vi "GrubbsTest.vi"(4 "Значимость":dbl, 6 "Исходные":dbl[](graph)) -> (0 "СКО":dbl, 1 "Среднее":dbl, 2 "Промахи":dbl[](array[numeric]), 3 "Обработанные":dbl[](graph))   [LabVIEW 2013]
uses:
  <vilib>/Analysis/NI_AALBase.lvlib
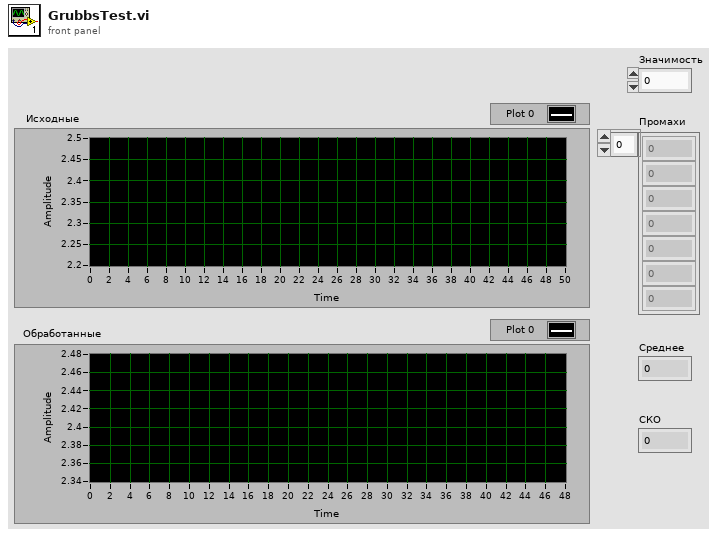
[diagram p1: front panel]
types:
  T1 = enum16{"Init", "GradeCount", "MissChecks", "fin"}
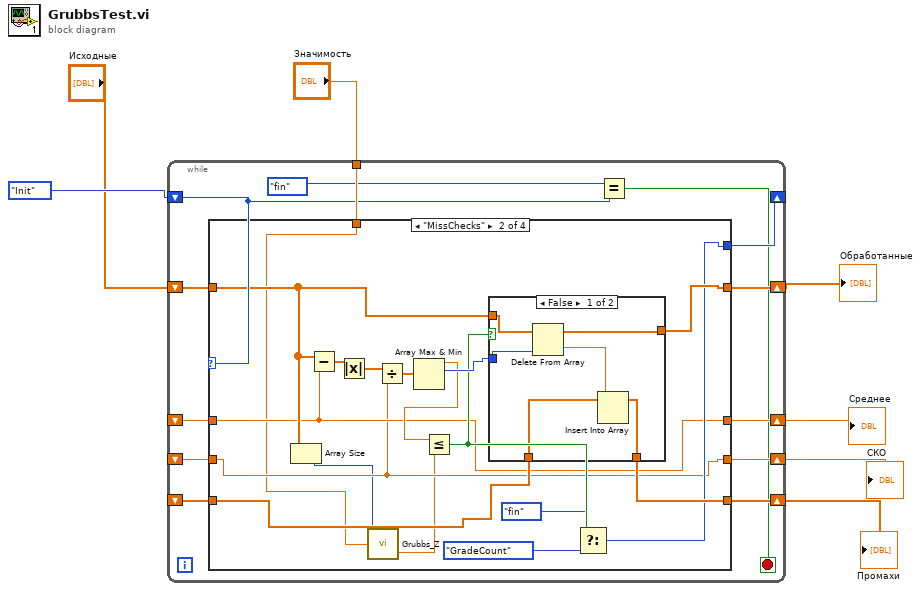
[diagram p0: block diagram]
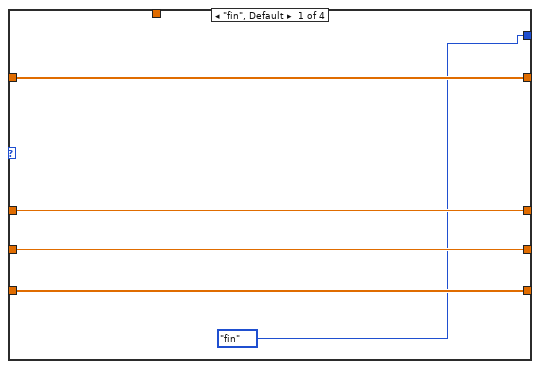
[diagram p2: hidden frame]
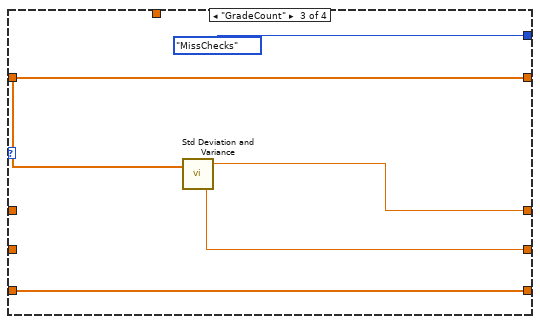
[diagram p4: hidden frame]
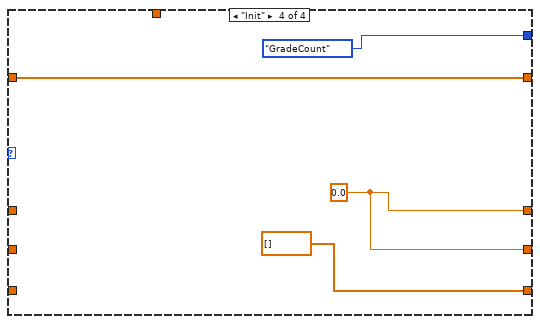
[diagram p5: hidden frame]
diagram:
  n1 = while {
    shift-right: [w20] -> _
    shift-left: T1."Init" -> [w9]
    tunnel: "Значимость" -> [w19]
    shift-right: [w14] -> w5
    shift-left: "Исходные" -> [w18]
    shift-right: [w17] -> w4
    shift-left: _ -> [w11]
    shift-right: [w16] -> w3
    shift-left: _ -> [w12]
    shift-right: [w15] -> w2
    shift-left: _ -> [w13]
    stop <- w10 stop-if-true
    n2 = case shown="\"MissChecks\"" w9 {
      tunnel: [T1."fin" w35 T1."MissChecks" T1."GradeCount"] -> w20
      tunnel: w19 -> [_ w26 _ _]
      tunnel: w18 -> [w22 w32 w55 w59]
      tunnel: [w23 w31 w54 w58] -> w17
      tunnel: [w24 w30 w56 w58] -> w16
      tunnel: [w25 w42 w53 dbl[] []] -> w15
      tunnel: [w22 w41 w55 w59] -> w14
      tunnel: w13 -> [w25 w34 w53 _]
      tunnel: w12 -> [w24 w30 _ _]
      tunnel: w11 -> [w23 w31 _ _]
      frame "fin", Default {
      }
      frame "MissChecks" {
        n3 = Array Size(array=w32) -> (size(s)=w28:i32)
        n4 = Subtract(x=w32, y=w31) -> (x-y=w33:dbl[])
        n5 = Absolute Value(x=w33) -> (abs(x)=w43:dbl[])
        n6 = call "Grubbs_Z.vi"("n"=w28, "q"=w26) -> ("G"=w27:dbl)  [unwired: 2 in]
        n7 = Divide(x=w43, y=w30) -> (x/y=w29:dbl[])
        n8 = Array Max & Min(array=w29) -> (max value=w39:dbl, max index (indices)=w40:i32)  [unwired: 2 out]
        n9 = Less Or Equal?(x=w39, y=w27) -> (x <= y?=w38:bool)
        n10 = case shown="False" w38 {
          tunnel: w32 -> [w48 w51]
          tunnel: [w45 w50] -> w42
          tunnel: [w47 w51] -> w41
          tunnel: w40 -> [w44 _]
          tunnel: w34 -> [w46 w50]
          frame False {
            n11 = Delete From Array(array=w48, index=w44) -> (deleted portion=w49:dbl, array with subset deleted=w47:dbl[])  [unwired: 1 in]
            n12 = Insert Into Array(array=w46, new element=w49) -> (w45:dbl[])  [unwired: 1 in]
          }
          frame True {
          }
        }
        n13 = Select(t=T1."fin", s=w38, f=T1."GradeCount") -> (s? t:f=w35:T1)
      }
      frame "GradeCount" {
        n14 = call <vilib>:"Std Deviation and Variance.vi"("X"=w55) -> ("mean"=w54:dbl, "standard deviation"=w56:dbl)  [unwired: 1 in, 1 out]
      }
      frame "Init" {
        w58 = 0.0
      }
    }
    n15 = Equal?(x=T1."fin", y=w9) -> (x = y?=w10:bool)
  }
  "Промахи" <- w2
  "Обработанные" <- w5
  "Среднее" <- w4
  "СКО" <- w3
